vi "Set Opposite Rule.vi"(11 "Rule in":T1) -> (3 "opposite rule":T1)   [LabVIEW 2023]
uses:
  Cluster_Rule.ctl
  ENUM_Compare.ctl
  ENUM_Value Type.ctl
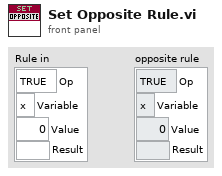
[diagram p1: front panel]
types:
  T1 = typedef "Cluster_Rule.ctl" = cluster{"Op":T2, "Variable":T3, "Value":i32, "Result":string}
  T2 = typedef "ENUM_Compare.ctl" = enum16{"TRUE", "<", ">", "<=", ">="}
  T3 = typedef "ENUM_Value Type.ctl" = enum16{"x", "m", "a", "s"}
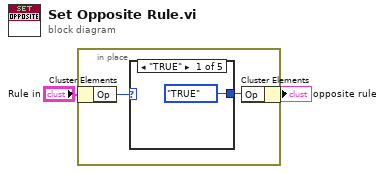
[diagram p0: block diagram]
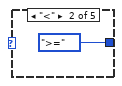
[diagram p2: hidden frame]
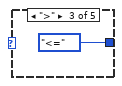
[diagram p3: hidden frame]
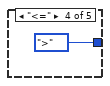
[diagram p4: hidden frame]
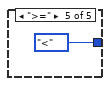
[diagram p5: hidden frame]
diagram:
  n1 = in-place {
    n2 = in-place-cluster #1("Rule in") -> ("Op"=w4:T2)
    n3 = case shown="\"TRUE\"" w4 {
      tunnel: [ENUM_Compare."TRUE" ("Op") ENUM_Compare.">=" ("Op") ENUM_Compare."<=" ("Op") ENUM_Compare.">" ("Op") ENUM_Compare."<" ("Op")] -> w3
      frame "TRUE" {
      }
      frame "<" {
      }
      frame ">" {
      }
      frame "<=" {
      }
      frame ">=" {
      }
    }
    n4 = in-place-cluster #1("Op"=w3) -> (→"opposite rule":T1)
  }
